vi "Initialization VI.vi"(8 "error in (no error)":errorcluster, 10 "Custom XML":string, 11 "Device Item Ref in":T1 format="%.0x") -> (0 "error out":errorcluster, 3 "Device Item Ref out":T1 format="%.0x")   [LabVIEW 2026, in "Nominal Core Streaming System Explorer.lvlib"]
uses:
  Nominal Core Streaming System Explorer.lvlib
  <vilib>/NI VeriStand/Custom Device API/Custom Device Item Ref.ctl
  <vilib>/NI VeriStand/Custom Device API/Set Item Property (U16).vi
  <vilib>/NI VeriStand/Custom Device API/Custom Device API.lvlib
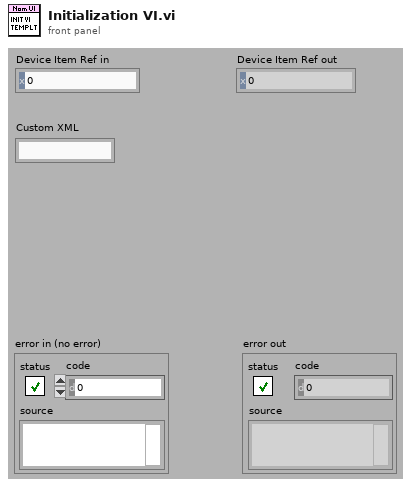
[diagram p1: front panel]
types:
  T1 = typedef "Custom Device API.lvlib/Custom Device Item Ref.ctl" = u64
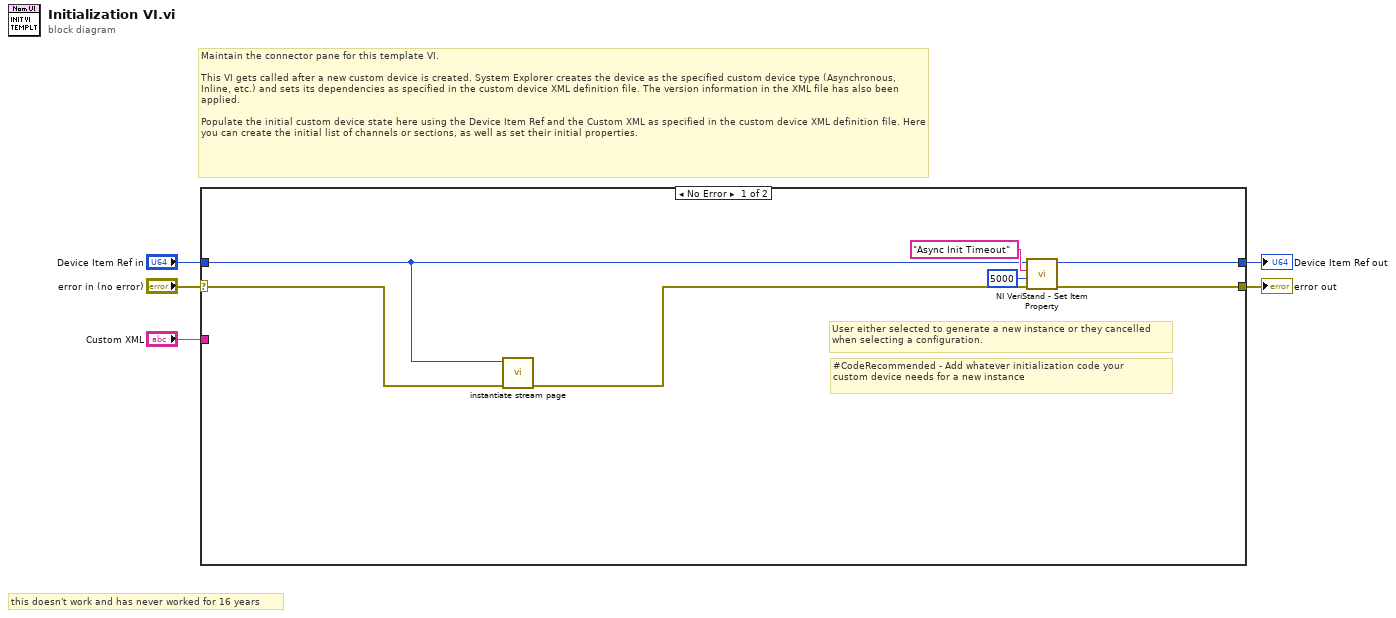
[diagram p0: block diagram]
diagram:
  # "this doesn't work and has never worked for 16 years"
  # "Maintain the connector pane for this template VI.\n\nThis VI gets called after a new custom device is created. System Explorer creates the device as the specified custom device type (Asynchronous, Inline, etc.) and sets its dependencies as specified in the custom device XML definition file. The version information in the XML file has also been applied.\n\nPopulate the initial custom device state here using the Device Item Ref and the Custom XML as specified in the custom device XML definition file. Here you can create the initial list of channels or sections, as well as set their initial properties."
  n1 = case shown="No Error" "error in (no error)" {
    selector: "error in (no error)" -> [w7 w14]
    tunnel: [w12 w14] -> w5
    tunnel: [w11 w13] -> w3
    tunnel: "Device Item Ref in" -> [w8 w13]
    tunnel: "Custom XML" -> [_ _]
    frame No Error {
      # "#CodeRecommended - Add whatever initialization code your\ncustom device needs for a new instance"
      # "User either selected to generate a new instance or they cancelled\nwhen selecting a configuration."
      n2 = call "instantiate stream page.vi"("error in (no error)"=w7, "stream"=w8) -> ("error out"=w6:errorcluster)  [unwired: 9 in]
      n3 = call-poly <vilib>:"NI VeriStand - Set Item Property.vi"("error in (no error)"=w6, "Value"=u16 5000, "Property Name"="Async Init Timeout", "Item Ref in"=w8) -> ("error out"=w12:errorcluster, "Item Ref out"=w11:T1)  [unwired: 5 in, 1 out]
    }
    frame Error {
    }
  }
  "error out" <- w5
  "Device Item Ref out" <- w3
